vi "array comb generator.vi"(0 "AO Vertical Range":dbl, 1 "Sampling Info in":cluster{"Fs":dbl, "#s":dbl}, 5 "Frequencies (Hz) in":dbl[](array[numeric]) format="%#_6p", 7 "number of bits":i16=16, 9 "Magnitude Initialization Vpp in":dbl[](array[numeric]), 11 "error in (no error)":errorcluster, 12 "Phases to maximize\ndestructive inter.":dbl[](array[numeric])) -> (3 "error out":errorcluster, 4 "Waveform Data":i16[](array[numeric]), 6 "Waveform Data 2":i16[](array[numeric]), 8 "Output Waveform Size":u32, 13 "signal out":waveform(dbl), 14 "signal out 2":waveform(dbl), 15 "Output Waveform Size 2":u32)   [LabVIEW 2020]
uses:
  <vilib>/measure/NI_MAPro.lvlib
panel:
  out "actual tone frequencies 2":dbl[](array[numeric]) format="%#_6p"
  out "actual tone frequencies":dbl[](array[numeric]) format="%#_6p"
  out "Waveform Graph 2":waveform(dbl)(graph)
  out "Waveform Graph":waveform(dbl)(graph)
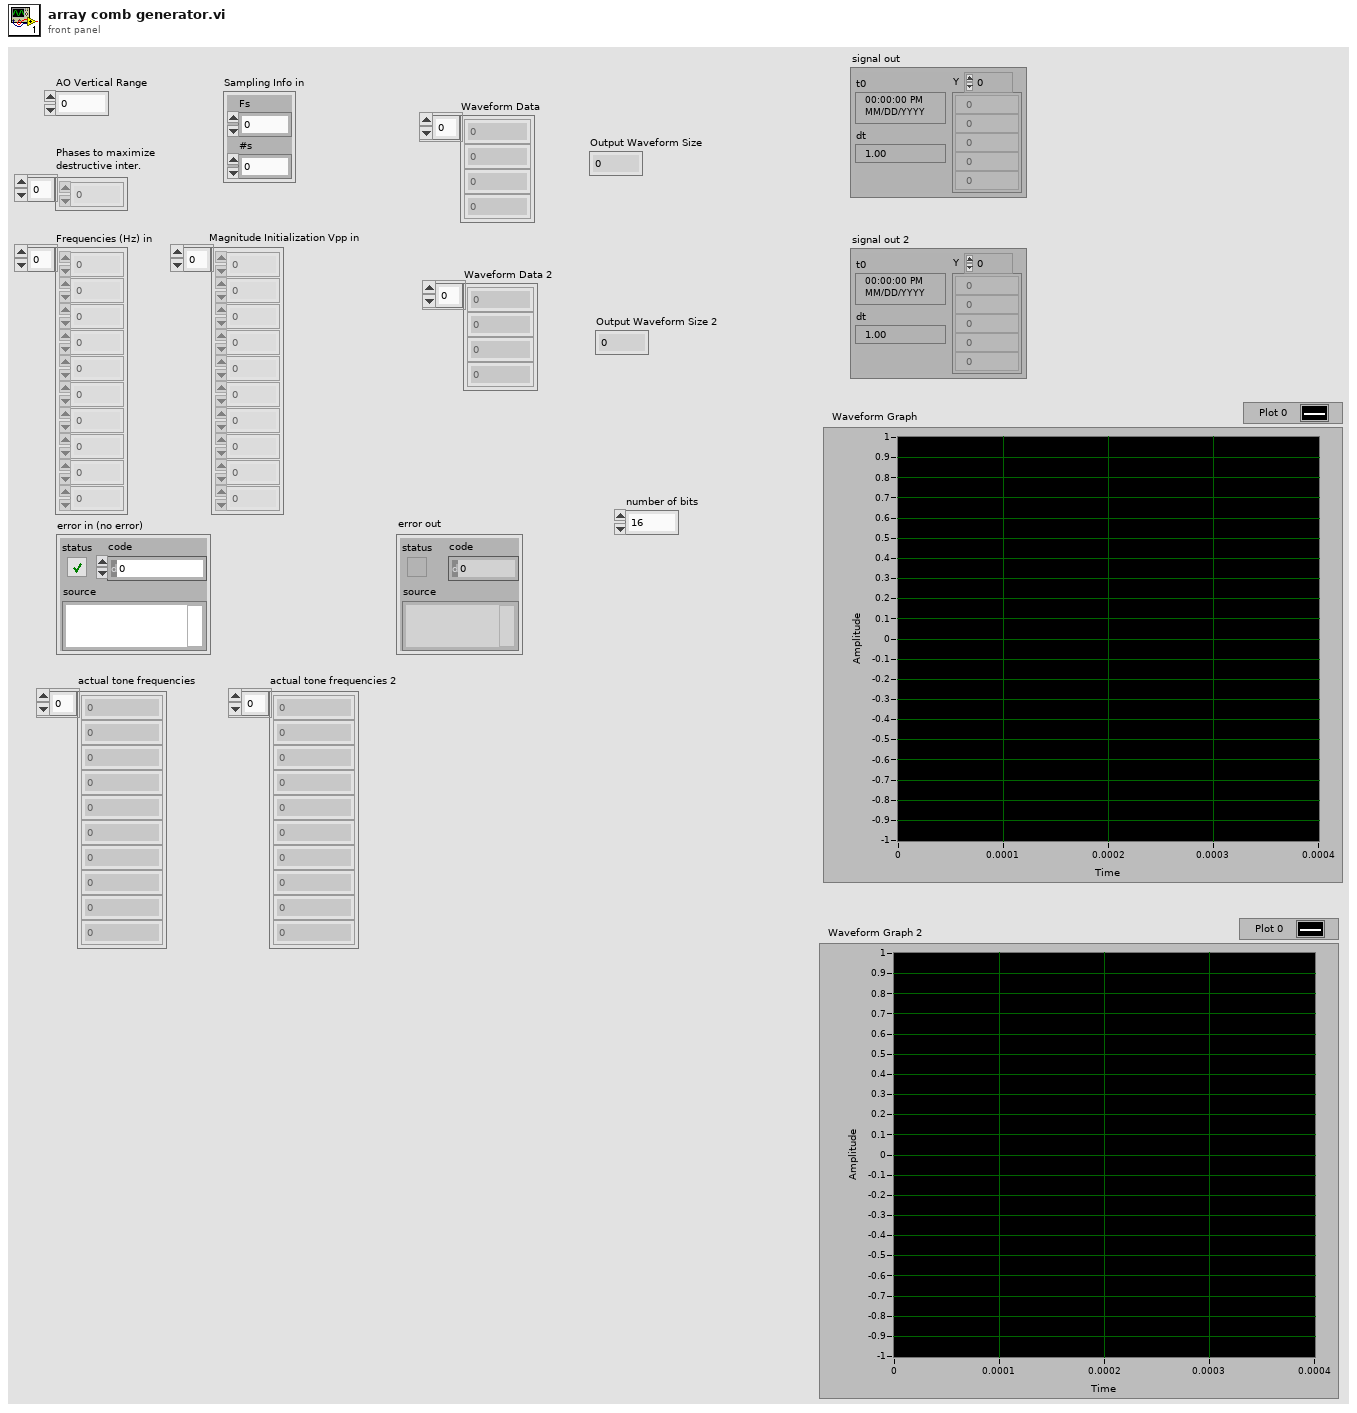
[diagram p1: front panel]
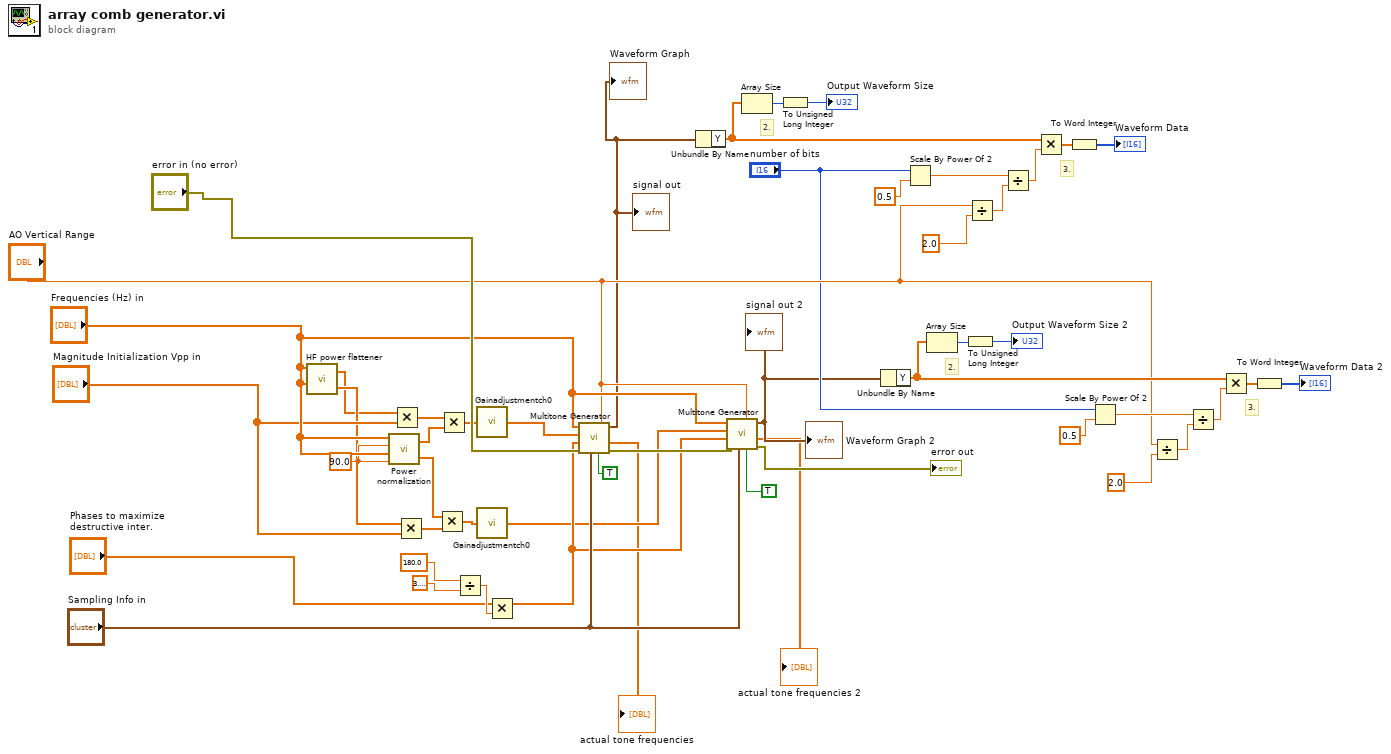
[diagram p0: block diagram]
diagram:
  w39 = 90.0 ("% of max CH 0")
  # "2."
  # "3."
  # "2."
  # "3."
  n1 = call "HF power flattener.vi"("CH 1 frequency"="Frequencies (Hz) in", "CH 0 frequency"="Frequencies (Hz) in") -> ("Normalized CH1"=w37:dbl[], "Normalized CH 0"=w33:dbl[])  [unwired: 2 in]
  n2 = call "Power normalization.vi"("% of max CH 1"=w39, "CH 1 frequency"="Frequencies (Hz) in", "% of max CH 0"=w39, "CH 0 frequency"="Frequencies (Hz) in") -> ("Normalized CH1"=w36:dbl[], "Normalized CH 0"=w30:dbl[])
  n3 = Multiply(x=w33, y="Magnitude Initialization Vpp in") -> (x*y=w31:dbl[])
  n4 = Multiply(x=w37, y="Magnitude Initialization Vpp in") -> (x*y=w35:dbl[])
  n5 = Multiply(x=w36, y=w35) -> (x*y=w34:dbl[])
  n6 = Multiply(x=w31, y=w30) -> (x*y=w32:dbl[])
  n7 = Divide(x=180.0, y=3.141592653589793) -> (x/y=w44:dbl)
  n8 = call "Gainadjustmentch0.vi"("Gain"=w32) -> ("Adjusted gain"=w40:dbl[])
  n9 = call "Gainadjustmentch0.vi"("Gain"=w34) -> ("Adjusted gain"=w46:dbl[])
  n10 = Multiply(x="Phases to maximize\ndestructive inter.", y=w44) -> (x*y=w47:dbl[])
  n11 = call <vilib>:"Multitone Generator.vi"("coerce frequencies?"=TRUE, "amplitude"="AO Vertical Range", "sampling info"="Sampling Info in", "error in (no error)"="error in (no error)", "tone phases"=w47, "tone amplitudes"=w40, "tone frequencies"="Frequencies (Hz) in") -> ("error out"=w50:errorcluster, "actual tone frequencies"=→"actual tone frequencies":dbl[], "signal out"=w5:waveform(dbl))  [unwired: 1 in, 1 out]
  "signal out" <- w5
  "Waveform Graph" <- w5
  n12 = Unbundle By Name(w5) -> ("Y"=w25:dbl[])
  n13 = call <vilib>:"Multitone Generator.vi"("coerce frequencies?"=TRUE, "amplitude"="AO Vertical Range", "sampling info"="Sampling Info in", "error in (no error)"=w50, "tone phases"=w47, "tone amplitudes"=w46, "tone frequencies"="Frequencies (Hz) in") -> ("error out"=→"error out":errorcluster, "actual tone frequencies"=→"actual tone frequencies 2":dbl[], "signal out"=w6:waveform(dbl))  [unwired: 1 in, 1 out]
  "signal out 2" <- w6
  "Waveform Graph 2" <- w6
  n14 = Array Size(array=w25) -> (size(s)=w29:i32)
  n15 = To Unsigned Long Integer(number=w29) -> (unsigned 32bit integer=→"Output Waveform Size":u32)
  n16 = Unbundle By Name(w6) -> ("Y"=w14:dbl[])
  n17 = Scale By Power Of 2(n="number of bits", x=0.5) -> (x*2^n=w26:dbl)
  n18 = Array Size(array=w14) -> (size(s)=w18:i32)
  n19 = To Unsigned Long Integer(number=w18) -> (unsigned 32bit integer=→"Output Waveform Size 2":u32)
  n20 = Divide(x="AO Vertical Range", y=2.0 ("x")) -> (x/y=w21:dbl)
  n21 = Divide(x=w26, y=w21) -> (x/y=w23:dbl)
  n22 = Multiply(x=w25, y=w23) -> (x*y=w28:dbl[])
  n23 = To Word Integer(number=w28) -> (16bit integer=→"Waveform Data":i16[])
  n24 = Scale By Power Of 2(n="number of bits", x=0.5) -> (x*2^n=w15:dbl)
  n25 = Divide(x="AO Vertical Range", y=2.0 ("x")) -> (x/y=w10:dbl)
  n26 = Divide(x=w15, y=w10) -> (x/y=w12:dbl)
  n27 = Multiply(x=w14, y=w12) -> (x*y=w17:dbl[])
  n28 = To Word Integer(number=w17) -> (16bit integer=→"Waveform Data 2":i16[])
